vi "Timestamp(s) with error-clusters.vi"(4 "Error In":errorcluster) -> (0 "Error Out":errorcluster, 3 "Time Stamp (sec)":timestamp)   [LabVIEW 2015, in "Timing.lvlib"]
uses:
  Timing.lvlib
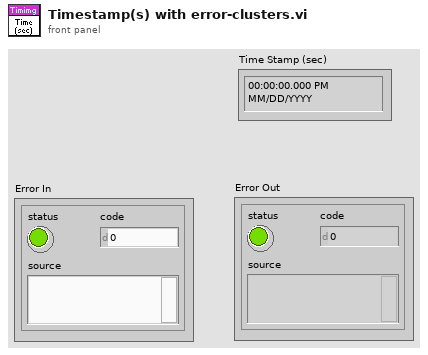
[diagram p1: front panel]
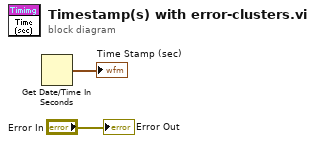
[diagram p0: block diagram]
diagram:
  n1 = Get Date/Time In Seconds() -> (seconds since 1Jan1904=→"Time Stamp (sec)":timestamp)
  "Error Out" <- "Error In"
